vi "Anritsu VNA Set Power.vi"(6 "Channel":i8=1 min=1 step=1, 7 "Anritsu VNA":T1, 8 "error in (no error)":errorcluster, 10 "Source Power, dBm (0.0)":dbl, 11 "VISA Resource Name":refnum<visa-resource-name>) -> (0 "error out":errorcluster, 3 "dup VISA Resource Name":refnum<visa-resource-name>)   [LabVIEW 2011]
doc: "This vi sets the power range. Only works on the HP 8753D."
uses:
  TypeDefs/Anritsu VNA Instrument Info.ctl
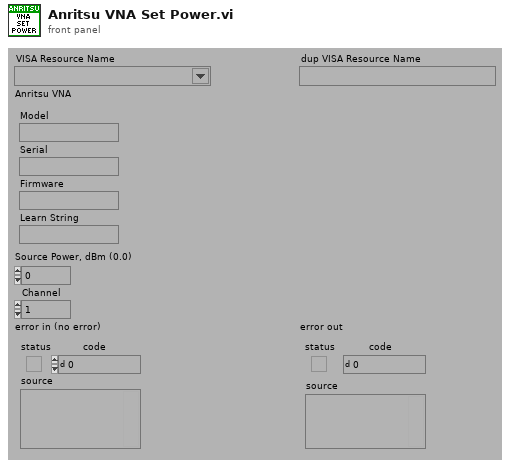
[diagram p1: front panel]
types:
  T1 = typedef "Anritsu VNA Instrument Info.ctl" = cluster{"Model":string, "Serial":string, "Firmware":string, "Learn String":string}
  T2 = typedef "Anritsu VNA Model.ctl" = enum16{"Not Supported", "37XXXX", "MS20XXX", "MS462XX", "MS464XX"}
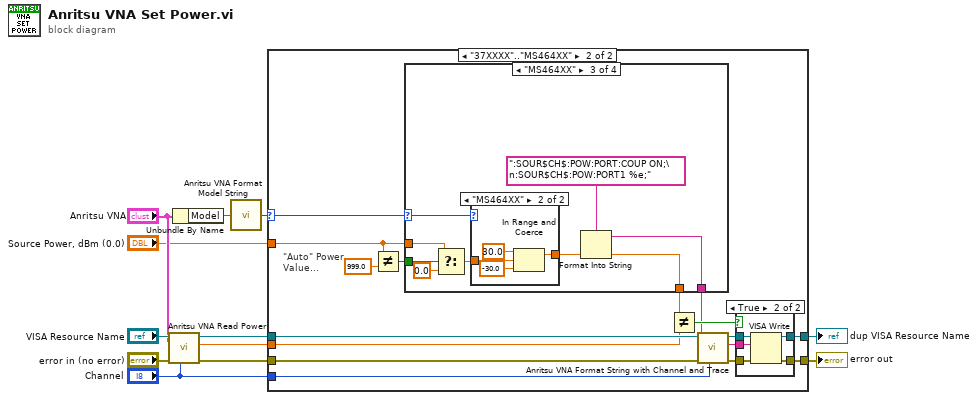
[diagram p0: block diagram]
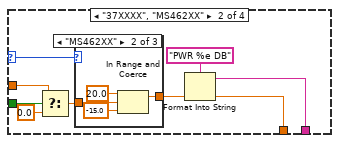
[diagram p4: hidden frame]
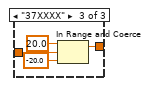
[diagram p6: hidden frame]
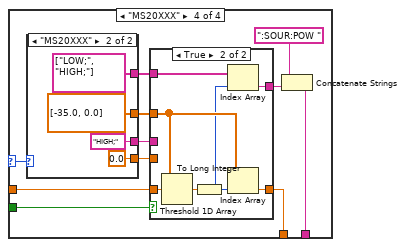
[diagram p8: hidden frame]
diagram:
  n1 = call "Anritsu VNA Read Power.vi"("Channel"="Channel", "Anritsu VNA"="Anritsu VNA", "error in (no error)"="error in (no error)", "VISA Resource Name"="VISA Resource Name") -> ("error out"=w9:errorcluster, "Source Power, dBm"=w6:dbl, "dup VISA Resource Name"=w7:refnum<visa-resource-name>)  [unwired: 5 out]
  n2 = Unbundle By Name("Anritsu VNA") -> ("Model"=w3:string)
  n3 = call "Anritsu VNA Format Model String.vi"("Model"=w3) -> ("Model"=w2:T2)
  n4 = case shown="\"37XXXX\"..\"MS464XX\"" w2 {
    selector: w2 -> [_ w18]
    tunnel: [w13 w28] -> w12
    tunnel: [w14 w27] -> w11
    tunnel: w9 -> [w13 w25]
    tunnel: w7 -> [w14 w24]
    tunnel: w6 -> [_ w23]
    tunnel: "Source Power, dBm (0.0)" -> [_ w19]
    tunnel: "Channel" -> [_ w15]
    frame "Not Supported" {
    }
    frame "37XXXX".."MS464XX" {
      # "\"Auto\" Power\nValue..."
      n5 = Not Equal?(x=w19, y=999.0) -> (x != y?=w20:bool)
      n6 = case shown="\"MS464XX\"" w18 {
        selector: w18 -> [_ w31 w47 w57]
        tunnel: [_ w30 w46 w64] -> w17
        tunnel: [_ w29 w45 w61] -> w21
        tunnel: w20 -> [_ w36 w52 w60]
        tunnel: w19 -> [_ w35 w51 w58]
        frame "Not Supported" {
        }
        frame "37XXXX", "MS462XX" {
          n7 = Select(t=w35, s=w36, f=0.0) -> (s? t:f=w33:dbl)
          n8 = case shown="\"MS462XX\"" w31 {
            tunnel: w33 -> [_ w40 w44]
            tunnel: [_ w37 w41] -> w29
            frame "Not Supported", "MS20XXX", "MS464XX" {
            }
            frame "MS462XX" {
              n9 = In Range and Coerce(upper limit=20.0, x=w40, lower limit=-15.0) -> (coerced(x)=w37:dbl)  [unwired: 1 out]
            }
            frame "37XXXX" {
              n10 = In Range and Coerce(upper limit=20.0, x=w44, lower limit=-20.0) -> (coerced(x)=w41:dbl)  [unwired: 1 out]
            }
          }
          n11 = Format Into String(format string="PWR %e DB", w29) -> (resulting string=w30:string)  [unwired: 2 in, 1 out]
        }
        frame "MS464XX" {
          n12 = Select(t=w51, s=w52, f=0.0) -> (s? t:f=w49:dbl)
          n13 = case shown="\"MS464XX\"" w47 {
            tunnel: w49 -> [_ w56]
            tunnel: [_ w53] -> w45
            frame "Not Supported".."MS462XX" {
            }
            frame "MS464XX" {
              n14 = In Range and Coerce(upper limit=30.0, x=w56, lower limit=-30.0) -> (coerced(x)=w53:dbl)  [unwired: 1 out]
            }
          }
          n15 = Format Into String(format string=":SOUR$CH$:POW:PORT:COUP ON;\n:SOUR$CH$:POW:PORT1 %e;", w45) -> (resulting string=w46:string)  [unwired: 2 in, 1 out]
        }
        frame "MS20XXX" {
          n16 = case shown="\"MS20XXX\"" w57 {
            tunnel: [_ dbl[] [-35.0, 0.0]] -> w67
            tunnel: [_ string[] ["LOW;", "HIGH;"]] -> w66
            tunnel: [_ "HIGH;"] -> w65
            tunnel: [_ 0.0] -> w62
            frame "Not Supported", "37XXXX", "MS462XX", "MS464XX" {
            }
            frame "MS20XXX" {
            }
          }
          n17 = case shown="True" w60 {
            tunnel: w67 -> [_ w79]
            tunnel: w66 -> [_ w78]
            tunnel: [w73 w77] -> w63
            tunnel: w65 -> [w73 _]
            tunnel: [w72 w76] -> w61
            tunnel: w62 -> [w72 _]
            tunnel: w58 -> [_ w75]
            frame False {
            }
            frame True {
              n18 = Threshold 1D Array(2:w75, 3:w79) -> (0:w80:dbl)  [unwired: 1 out]
              n19 = To Long Integer(number=w80) -> (32bit integer=w74:i32)
              n20 = Index Array(array=w78, index=w74) -> (element=w77:string)
              n21 = Index Array(array=w79, index=w74) -> (element=w76:dbl)
            }
          }
          n22 = Concatenate Strings(":SOUR:POW ", w63) -> (w64:string)
        }
      }
      n23 = Not Equal?(x=w21, y=w23) -> (x != y?=w22:bool)
      n24 = call "Anritsu VNA Format String with Channel and Trace.vi"("Channel"=w15, "String"=w17) -> ("String Out"=w16:string)  [unwired: 1 in, 6 out]
      n25 = case shown="True" w22 {
        tunnel: [w81 w87] -> w28
        tunnel: [w82 w86] -> w27
        tunnel: w16 -> [_ w85]
        tunnel: w25 -> [w81 w84]
        tunnel: w24 -> [w82 w83]
        frame False {
        }
        frame True {
          n26 = VISA Write(VISA resource name=w83, write buffer=w85, error in (no error)=w84) -> (VISA resource name out=w86:refnum<visa-resource-name>, error out=w87:errorcluster)  [unwired: 1 out]
        }
      }
    }
  }
  "dup VISA Resource Name" <- w11
  "error out" <- w12
